vi "init.vi"(8 "error in (no error)":errorcluster) -> (0 "error out":errorcluster, 3 "objects":T1)   [LabVIEW 2025]
uses:
  Classes/Processor/Processor.lvclass
  <vilib>/Utility/sysdir.llb/System Directory Type.ctl
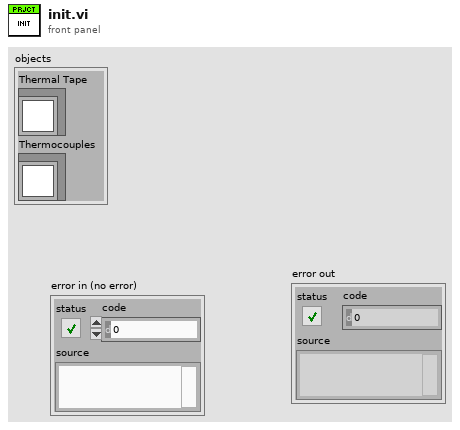
[diagram p1: front panel]
types:
  T1 = cluster{"Thermal Tape":refnum<class "Processor.lvclass">, "Thermocouples":refnum<class "Processor.lvclass">}
  T2 = typedef "System Directory Type.ctl" = i32
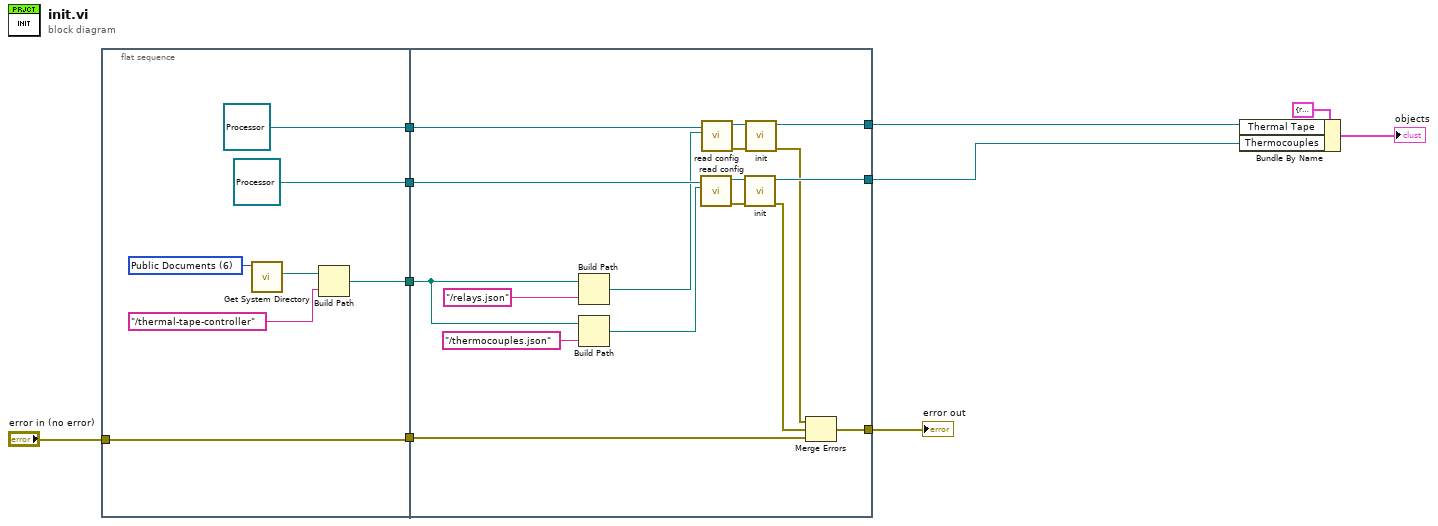
[diagram p0: block diagram]
diagram:
  n1 = flat-sequence {
    tunnel: [refnum<class "Processor.lvclass"> refnum ("Processor.lvclass")] -> w8
    tunnel: [refnum<class "Processor.lvclass"> refnum ("Processor.lvclass")] -> w7
    tunnel: [w12] -> w4
    tunnel: "error in (no error)" -> [w11]
    tunnel: [w11] -> w2
    tunnel: w8 -> [w29]
    tunnel: w7 -> [w30]
    tunnel: [w28] -> w6
    tunnel: [w27] -> w5
    tunnel: w4 -> [w25]
    tunnel: w2 -> [w19]
    tunnel: [w18] -> w1
    frame #0 {
      w15 = T2 6 items=["User Home"=0, "User Desktop"=1, "User Documents"=2, "User Application Data"=3, "User Preferences"=4, "User Temporary"=5, "Public Documents"=6, "Public Application Data"=7, "Public Preferences"=8, "Public Cache"=13, "System Core Libraries"=9, "System Installed Libraries"=10, "Application Files"=11, "Boot Volume Root"=12] ("system directory type")
      n2 = call <vilib>:"Get System Directory.vi"("system directory type"=w15) -> ("system directory"=w14:path)  [unwired: 10 in]
      n3 = Build Path(base path=w14, name or relative path="/thermal-tape-controller") -> (appended path=w12:path)
    }
    frame #1 {
      n4 = Build Path(base path=w25, name or relative path="/relays.json") -> (appended path=w23:path)
      n5 = Build Path(base path=w25, name or relative path="/thermocouples.json") -> (appended path=w22:path)
      n6 = call-dynamic "read config.vi"("config file path"=w22, "Processor in"=w30) -> ("error out"=w33:errorcluster, "Processor out"=w34:refnum<class "Processor.lvclass">)  [unwired: 8 in]
      n7 = call-dynamic "read config.vi"("config file path"=w23, "Processor in"=w29) -> ("error out"=w32:errorcluster, "Processor out"=w31:refnum<class "Processor.lvclass">)  [unwired: 8 in]
      n8 = call-dynamic "init.vi"("error in (no error)"=w33, "Processor in"=w34) -> ("error out"=w20:errorcluster, "Processor out"=w28:refnum<class "Processor.lvclass">)  [unwired: 8 in]
      n9 = call-dynamic "init.vi"("error in (no error)"=w32, "Processor in"=w31) -> ("error out"=w21:errorcluster, "Processor out"=w27:refnum<class "Processor.lvclass">)  [unwired: 8 in]
      n10 = Merge Errors(w21, w20, w19) -> (w18:errorcluster)
    }
  }
  n11 = Bundle By Name(cluster=T1 {"Thermal Tape"=refnum, "Thermocouples"=refnum}, "Thermal Tape"=w5, "Thermocouples"=w6) -> (→"objects":T1)
  "error out" <- w1
